vi "TestDebug.vi"() -> ()   [LabVIEW 2023]
uses:
  Plugin/RMX41XPowerSupply/RMX41XPowerSupply.lvclass
panel:
  out "element 5":string
  out "element 4":string
  out "element 3":string
  out "element 2":string
  out "element":string
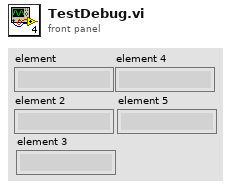
[diagram p1: front panel]
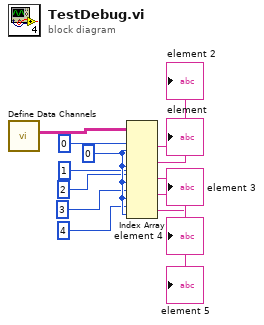
[diagram p0: block diagram]
diagram:
  w11 = 0 ("disabled index (col)")
  n1 = call "Define Data Channels.vi"() -> ("Tag Consumer Channels"=w12:string[][])  [unwired: 8 in, 3 out]
  n2 = Index Array(array=w12, index (row) #1=0 ("disabled index (row)"), index (col) #1=w11, index (row) #2=1 ("disabled index (row)"), index (col) #2=w11, index (row) #3=2 ("disabled index (row)"), index (col) #3=w11, index (row) #4=3 ("disabled index (row)"), index (col) #4=w11, index (row) #5=4 ("disabled index (row)"), index (col) #5=w11) -> (element #1=→"element":string, element #2=→"element 2":string, element #3=→"element 3":string, element #4=→"element 4":string, element #5=→"element 5":string)
